vi "BuildRunScript.vi"(8 "ErrorArray":errorcluster[](array[cluster]), 11 "Bus":refnum<class "Bus.lvclass">) -> (0 "ErrorArray":errorcluster[](array[cluster]), 2 "Script":string[](array[string]), 3 "Bus":refnum<class "Bus.lvclass">)   [LabVIEW 2014, in "Bus_class.lvlib" / "Bus.lvclass"]
uses:
  Bus.lvclass
  Modules/EventModule/PublicAPI/Arguments/Broadcasts/clErrorRpt.ctl
  <vilib>/Utility/error.llb/Error Cluster From Error Code.vi
  <vilib>/ErrorRing/Error Ring.xnode
  Modules/EventModule/EventModule.lvlib
  <userlib>/NIST/NISTErrorLib/NISTErrorLib.lvlib
  Modules/PmuImpairModule/PmuImpairModule.lvlib
  Modules/NetworkImpairmentModule/NetworkImpairmentModule.lvlib
  Modules/FlagImpairModule/FlagImpairModule.lvlib
  Modules/OutputToFileModule/OutputToFileModule.lvlib
  Modules/AppModule/AppModule.lvlib
  Modules/AppPlugins/AppPluginBaseClass/AppPluginsBase.lvclass
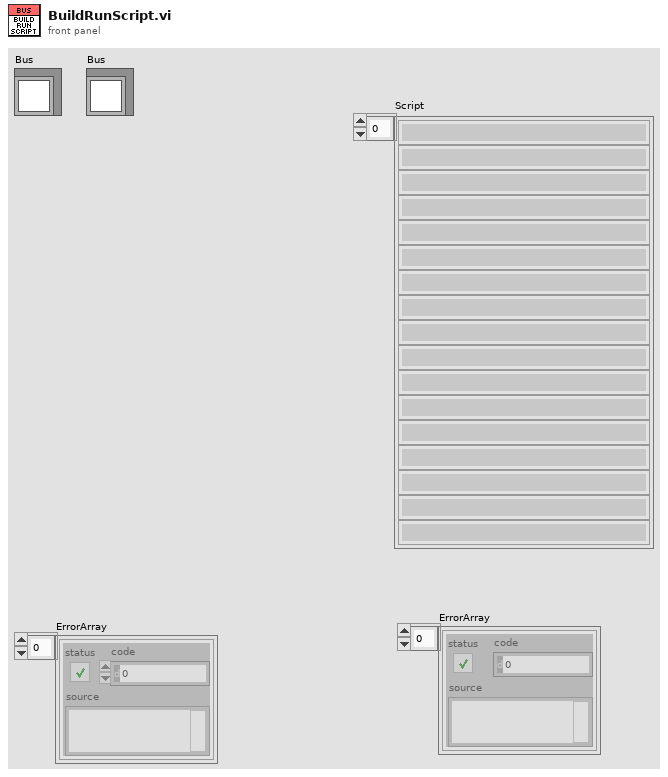
[diagram p1: front panel]
types:
  T1 = typedef "EventModule.lvlib/clErrorRpt.ctl" = cluster{"error":errorcluster, "AdditionalInfo":string}
  T2 = typedef "EventModule.lvlib/clBroadcastEvents.ctl" = cluster{"DidInit":refnum<user-event>, "StatusUpdate":refnum<user-event>, "ErrorReport":refnum<user-event>, "DidStop":refnum<user-event>, "ReadEvtConfig":refnum<user-event>, "ReadTimeArray":refnum<user-event>, "ReadEvtParams":refnum<user-event>, "GetEvtReportArray":refnum<user-event>, "ReadPathToPlugin":refnum<user-event>, "GetEvtSignal":refnum<user-event>, "ReadBusNumber":refnum<user-event>}
  T3 = typedef "PmuImpairModule.lvlib/clBroadcastEvents.ctl" = cluster{"DidInit":refnum<user-event>, "StatusUpdate":refnum<user-event>, "ErrorReport":refnum<user-event>, "DidStop":refnum<user-event>, "ImpairConfig":refnum<user-event>, "ImpairParams":refnum<user-event>, "ImpairReports":refnum<user-event>, "PathToPlugin":refnum<user-event>, "BusNumber":refnum<user-event>}
  T4 = typedef "NetworkImpairmentModule.lvlib/clBroadcastEvents.ctl" = cluster{"DidInit":refnum<user-event>, "StatusUpdate":refnum<user-event>, "ErrorReport":refnum<user-event>, "DidStop":refnum<user-event>, "ReadNetImpParams":refnum<user-event>, "ReadLossThreshold":refnum<user-event>, "GetNetworkTime":refnum<user-event>, "GetPktLoss":refnum<user-event>, "ReadPathToPlugin":refnum<user-event>}
  T5 = typedef "FlagImpairModule.lvlib/clBroadcastEvents.ctl" = cluster{"DidInit":refnum<user-event>, "StatusUpdate":refnum<user-event>, "ErrorReport":refnum<user-event>, "DidStop":refnum<user-event>, "ReadFlagImpairConfig":refnum<user-event>, "ReadPluginINIFilePath":refnum<user-event>, "ReadFlagImpairParams":refnum<user-event>, "ReadTimeArray":refnum<user-event>, "GetFlagImpairment":refnum<user-event>}
  T6 = typedef "OutputToFileModule.lvlib/clBroadcastEvents.ctl" = cluster{"DidInit":refnum<user-event>, "StatusUpdate":refnum<user-event>, "ErrorReport":refnum<user-event>, "DidStop":refnum<user-event>, "PathToPlugin":refnum<user-event>, "PmuConfig":refnum<user-event>, "OutputPath":refnum<user-event>}
  T7 = typedef "AppModule.lvlib/clBroadcastEvents.ctl" = cluster{"DidInit":refnum<user-event>, "StatusUpdate":refnum<user-event>, "ErrorReport":refnum<user-event>, "DidStop":refnum<user-event>, "PathToINI":refnum<user-event>, "InputData":refnum<user-event>, "OutputData":refnum<user-event>, "BcAppInfo":refnum<user-event>, "ConfigData":refnum<user-event>}
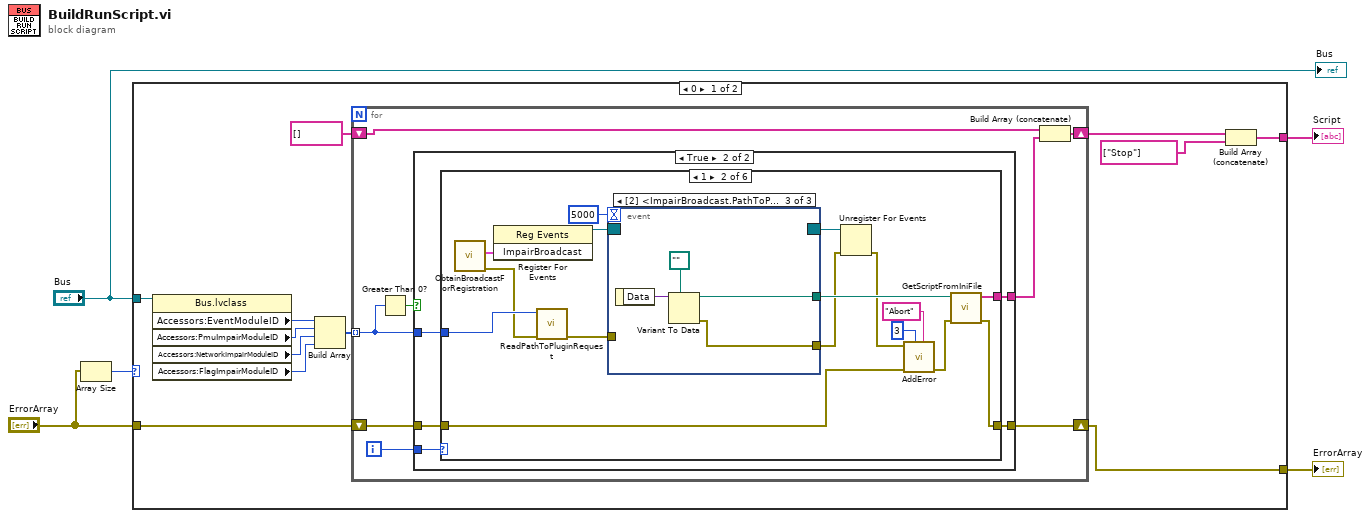
[diagram p0: block diagram]
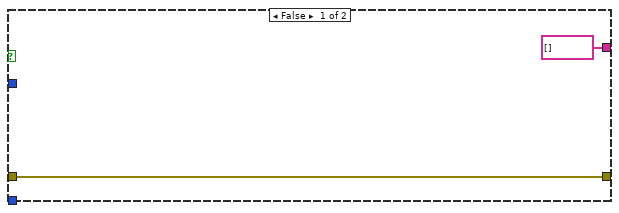
[diagram p2: hidden frame]
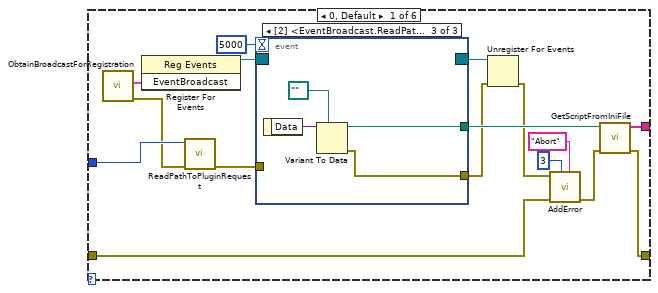
[diagram p3: hidden frame]
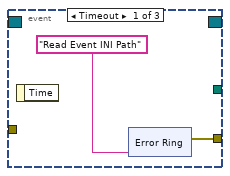
[diagram p4: hidden frame]
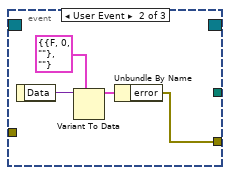
[diagram p5: hidden frame]
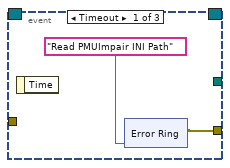
[diagram p6: hidden frame]
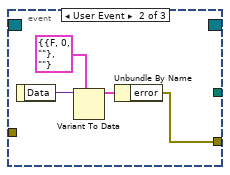
[diagram p7: hidden frame]
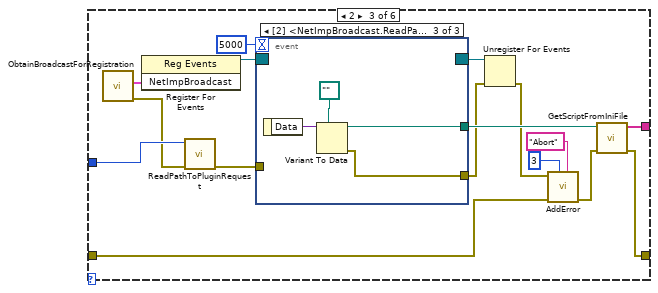
[diagram p8: hidden frame]
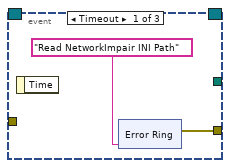
[diagram p9: hidden frame]
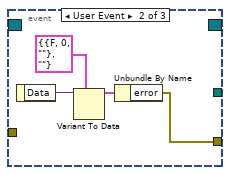
[diagram p10: hidden frame]
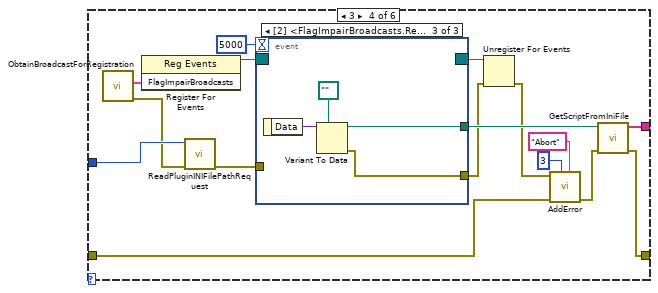
[diagram p11: hidden frame]
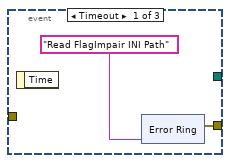
[diagram p12: hidden frame]
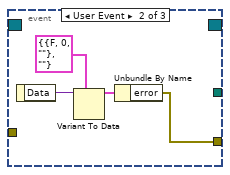
[diagram p13: hidden frame]
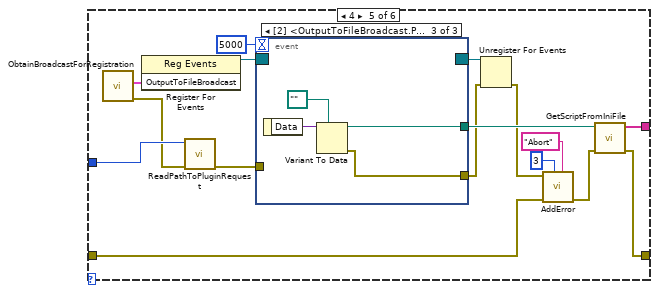
[diagram p14: hidden frame]
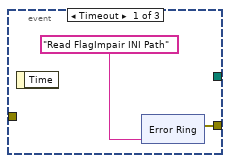
[diagram p15: hidden frame]
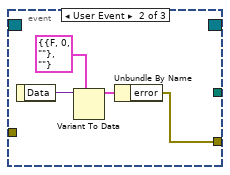
[diagram p16: hidden frame]
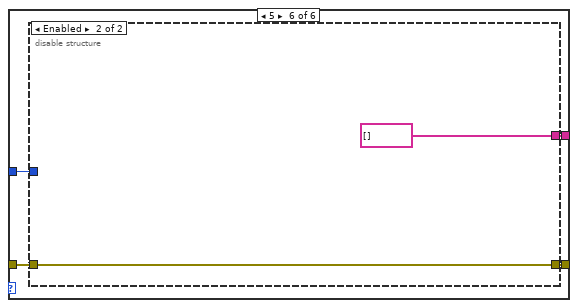
[diagram p17: hidden frame]
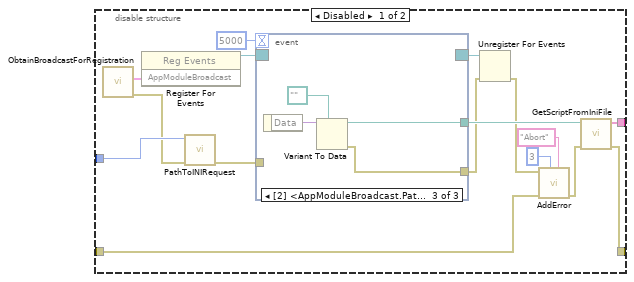
[diagram p18: hidden frame]
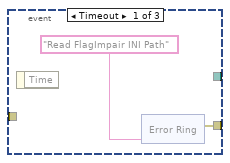
[diagram p19: hidden frame]
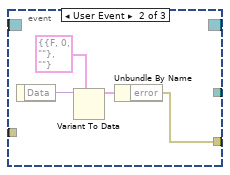
[diagram p20: hidden frame]
diagram:
  n1 = Array Size(array="ErrorArray") -> (size(s)=w5:i32)
  n2 = case shown="0" w5 {
    tunnel: "ErrorArray" -> [w10 w237]
    tunnel: [w8 w237] -> w3
    tunnel: [w17 _] -> w2
    tunnel: "Bus" -> [w6 _]
    frame 0 {
      n3 = property class="Bus.lvclass"(reference=w6) -> ("Accessors:EventModuleID"=w15:i32, "Accessors:PmuImpairModuleID"=w14:i32, "Accessors:NetworkImpairModuleID"=w13:i32, "Accessors:FlagImpairModuleID"=w12:i32)  [unwired: 1 in, 2 out]
      n4 = Build Array(w15, w14, w13, w12) -> (w11:i32[])
      n5 = for {
        tunnel: w11 -> [w18] mode=indexing
        shift-right: [w23] -> w8
        shift-left: w10 -> [w24]
        shift-right: [w21] -> w7
        shift-left: string[] [] -> [w20]
        i -> [w25]
        n6 = Greater Than 0?(x=w18) -> (x > 0?=w19:bool)
        n7 = case shown="True" w19 {
          tunnel: w25 -> [_ w32]
          tunnel: w18 -> [_ w31]
          tunnel: w24 -> [w26 w30]
          tunnel: [w26 w29] -> w23
          tunnel: [string[] [] ("Script") w28] -> w22
          frame False {
          }
          frame True {
            n8 = case shown="1" w32 {
              tunnel: w31 -> [w48 w81 w114 w147 w180 w201]
              tunnel: w30 -> [w38 w71 w104 w137 w170 w200]
              tunnel: [w37 w70 w103 w136 w169 w199] -> w29
              tunnel: [w36 w69 w102 w135 w168 w198] -> w28
              frame 0, Default {
                n9 = call "ObtainBroadcastForRegistration.vi"() -> ("error out"=w43:errorcluster, "EventBroadcast"=w47:T2)  [unwired: 10 in]
                n10 = register-events(w47) -> (reference out=w46:refnum<event-registration>)  [unwired: 2 in, 1 out]
                n11 = call "ReadPathToPluginRequest.vi"("error in (no error)"=w43, "ModuleID"=w48) -> ("error out"=w44:errorcluster)  [unwired: 9 in]
                n12 = event shown="[2] <EventBroadcast.ReadPathToPlugin>: User Event" {
                  selector: w46 -> [_ _ _]
                  dyn-events: [_ _ _] -> w35
                  timeout: 5000 -> [_ _ _]
                  tunnel: [w50 w58 w63] -> w34
                  tunnel: w44 -> [_ _ _]
                  tunnel: [_ _ w62] -> w42
                  event Timeout {
                    n13 = event-data() -> ()  [unwired: 1 in, 1 out]
                    n14 = xnode "Error Ring"("parameter 0"="Read Event INI Path") -> ("error out"=w50:errorcluster)
                  }
                  event User Event {
                    n15 = event-data() -> ("Data"=w61:variant)  [unwired: 1 in]
                    n16 = Variant To Data(type=T1 {"error"={"status"=FALSE, "code"=0, "source"=""}, "AdditionalInfo"=""} ("Cluster"), Variant=w61) -> (data=w59:T1)  [unwired: 1 in, 1 out]
                    n17 = Unbundle By Name(w59) -> ("error"=w58:errorcluster)
                  }
                  event User Event {
                    n18 = event-data() -> ("Data"=w65:variant)  [unwired: 1 in]
                    n19 = Variant To Data(type=path "", Variant=w65) -> (data=w62:path, error out=w63:errorcluster)  [unwired: 1 in]
                  }
                }
                n20 = Unregister For Events(event registration refnum=w35, error in=w34) -> (error out=w33:errorcluster)
                n21 = call <userlib>:"AddError.vi"("Severity"="Abort" ("String"), "Priority"=u8 3, "ErrorArray"=w38, "error in (no error)"=w33) -> ("ErrorArray"=w39:errorcluster[])  [unwired: 6 in, 1 out]
                n22 = call "GetScriptFromIniFile.vi"("ErrorArray"=w39, "Path"=w42) -> ("ErrorArray"=w37:errorcluster[], "Script"=w36:string[])  [unwired: 8 in]
              }
              frame 1 {
                n23 = call "ObtainBroadcastForRegistration.vi"() -> ("error out"=w76:errorcluster, "ImpairBroadcast"=w80:T3)  [unwired: 10 in]
                n24 = register-events(w80) -> (reference out=w79:refnum<event-registration>)  [unwired: 2 in, 1 out]
                n25 = call "ReadPathToPluginRequest.vi"("error in (no error)"=w76, "ModuleID"=w81) -> ("error out"=w77:errorcluster)  [unwired: 9 in]
                n26 = event shown="[2] <ImpairBroadcast.PathToPlugin>: User Event" {
                  selector: w79 -> [_ _ _]
                  dyn-events: [_ _ _] -> w68
                  timeout: 5000 -> [_ _ _]
                  tunnel: [w83 w91 w96] -> w67
                  tunnel: w77 -> [_ _ _]
                  tunnel: [_ _ w95] -> w75
                  event Timeout {
                    n27 = event-data() -> ()  [unwired: 1 in, 1 out]
                    n28 = xnode "Error Ring"("parameter 0"="Read PMUImpair INI Path") -> ("error out"=w83:errorcluster)
                  }
                  event User Event {
                    n29 = event-data() -> ("Data"=w94:variant)  [unwired: 1 in]
                    n30 = Variant To Data(type=T1 {"error"={"status"=FALSE, "code"=0, "source"=""}, "AdditionalInfo"=""} ("Cluster"), Variant=w94) -> (data=w92:T1)  [unwired: 1 in, 1 out]
                    n31 = Unbundle By Name(w92) -> ("error"=w91:errorcluster)
                  }
                  event User Event {
                    n32 = event-data() -> ("Data"=w98:variant)  [unwired: 1 in]
                    n33 = Variant To Data(type=path "", Variant=w98) -> (data=w95:path, error out=w96:errorcluster)  [unwired: 1 in]
                  }
                }
                n34 = Unregister For Events(event registration refnum=w68, error in=w67) -> (error out=w66:errorcluster)
                n35 = call <userlib>:"AddError.vi"("Severity"="Abort" ("String"), "Priority"=u8 3, "ErrorArray"=w71, "error in (no error)"=w66) -> ("ErrorArray"=w72:errorcluster[])  [unwired: 6 in, 1 out]
                n36 = call "GetScriptFromIniFile.vi"("ErrorArray"=w72, "Path"=w75) -> ("ErrorArray"=w70:errorcluster[], "Script"=w69:string[])  [unwired: 8 in]
              }
              frame 2 {
                n37 = call "ObtainBroadcastForRegistration.vi"() -> ("error out"=w109:errorcluster, "NetImpBroadcast"=w113:T4)  [unwired: 10 in]
                n38 = register-events(w113) -> (reference out=w112:refnum<event-registration>)  [unwired: 2 in, 1 out]
                n39 = call "ReadPathToPluginRequest.vi"("error in (no error)"=w109, "ModuleID"=w114) -> ("error out"=w110:errorcluster)  [unwired: 9 in]
                n40 = event shown="[2] <NetImpBroadcast.ReadPathToPlugin>: User Event" {
                  selector: w112 -> [_ _ _]
                  dyn-events: [_ _ _] -> w101
                  timeout: 5000 -> [_ _ _]
                  tunnel: [w116 w124 w129] -> w100
                  tunnel: w110 -> [_ _ _]
                  tunnel: [_ _ w128] -> w108
                  event Timeout {
                    n41 = event-data() -> ()  [unwired: 1 in, 1 out]
                    n42 = xnode "Error Ring"("parameter 0"="Read NetworkImpair INI Path") -> ("error out"=w116:errorcluster)
                  }
                  event User Event {
                    n43 = event-data() -> ("Data"=w127:variant)  [unwired: 1 in]
                    n44 = Variant To Data(type=T1 {"error"={"status"=FALSE, "code"=0, "source"=""}, "AdditionalInfo"=""} ("Cluster"), Variant=w127) -> (data=w125:T1)  [unwired: 1 in, 1 out]
                    n45 = Unbundle By Name(w125) -> ("error"=w124:errorcluster)
                  }
                  event User Event {
                    n46 = event-data() -> ("Data"=w131:variant)  [unwired: 1 in]
                    n47 = Variant To Data(type=path "", Variant=w131) -> (data=w128:path, error out=w129:errorcluster)  [unwired: 1 in]
                  }
                }
                n48 = Unregister For Events(event registration refnum=w101, error in=w100) -> (error out=w99:errorcluster)
                n49 = call <userlib>:"AddError.vi"("Severity"="Abort" ("String"), "Priority"=u8 3, "ErrorArray"=w104, "error in (no error)"=w99) -> ("ErrorArray"=w105:errorcluster[])  [unwired: 6 in, 1 out]
                n50 = call "GetScriptFromIniFile.vi"("ErrorArray"=w105, "Path"=w108) -> ("ErrorArray"=w103:errorcluster[], "Script"=w102:string[])  [unwired: 8 in]
              }
              frame 3 {
                n51 = call "ObtainBroadcastForRegistration.vi"() -> ("error out"=w142:errorcluster, "FlagImpairBroadcasts"=w146:T5)  [unwired: 10 in]
                n52 = register-events(w146) -> (reference out=w145:refnum<event-registration>)  [unwired: 2 in, 1 out]
                n53 = call "ReadPluginINIFilePathRequest.vi"("error in (no error)"=w142, "ModuleID"=w147) -> ("error out"=w143:errorcluster)  [unwired: 9 in]
                n54 = event shown="[2] <FlagImpairBroadcasts.ReadPluginINIFilePath>: User Event" {
                  selector: w145 -> [_ _ _]
                  dyn-events: [_ _ _] -> w134
                  timeout: 5000 -> [_ _ _]
                  tunnel: [w149 w157 w162] -> w133
                  tunnel: w143 -> [_ _ _]
                  tunnel: [_ _ w161] -> w141
                  event Timeout {
                    n55 = event-data() -> ()  [unwired: 1 in, 1 out]
                    n56 = xnode "Error Ring"("parameter 0"="Read FlagImpair INI Path") -> ("error out"=w149:errorcluster)
                  }
                  event User Event {
                    n57 = event-data() -> ("Data"=w160:variant)  [unwired: 1 in]
                    n58 = Variant To Data(type=T1 {"error"={"status"=FALSE, "code"=0, "source"=""}, "AdditionalInfo"=""} ("Cluster"), Variant=w160) -> (data=w158:T1)  [unwired: 1 in, 1 out]
                    n59 = Unbundle By Name(w158) -> ("error"=w157:errorcluster)
                  }
                  event User Event {
                    n60 = event-data() -> ("Data"=w164:variant)  [unwired: 1 in]
                    n61 = Variant To Data(type=path "", Variant=w164) -> (data=w161:path, error out=w162:errorcluster)  [unwired: 1 in]
                  }
                }
                n62 = Unregister For Events(event registration refnum=w134, error in=w133) -> (error out=w132:errorcluster)
                n63 = call <userlib>:"AddError.vi"("Severity"="Abort" ("String"), "Priority"=u8 3, "ErrorArray"=w137, "error in (no error)"=w132) -> ("ErrorArray"=w138:errorcluster[])  [unwired: 6 in, 1 out]
                n64 = call "GetScriptFromIniFile.vi"("ErrorArray"=w138, "Path"=w141) -> ("ErrorArray"=w136:errorcluster[], "Script"=w135:string[])  [unwired: 8 in]
              }
              frame 4 {
                n65 = call "ObtainBroadcastForRegistration.vi"() -> ("error out"=w175:errorcluster, "OutputToFileBroadcast"=w179:T6)  [unwired: 10 in]
                n66 = register-events(w179) -> (reference out=w178:refnum<event-registration>)  [unwired: 2 in, 1 out]
                n67 = call "ReadPathToPluginRequest.vi"("error in (no error)"=w175, "ModuleID"=w180) -> ("error out"=w176:errorcluster)  [unwired: 9 in]
                n68 = event shown="[2] <OutputToFileBroadcast.PathToPlugin>: User Event" {
                  selector: w178 -> [_ _ _]
                  dyn-events: [_ _ _] -> w167
                  timeout: 5000 -> [_ _ _]
                  tunnel: [w182 w190 w196] -> w166
                  tunnel: w176 -> [_ _ _]
                  tunnel: [_ _ w194] -> w174
                  event Timeout {
                    n69 = event-data() -> ()  [unwired: 1 in, 1 out]
                    n70 = xnode "Error Ring"("parameter 0"="Read FlagImpair INI Path") -> ("error out"=w182:errorcluster)
                  }
                  event User Event {
                    n71 = event-data() -> ("Data"=w193:variant)  [unwired: 1 in]
                    n72 = Variant To Data(type=T1 {"error"={"status"=FALSE, "code"=0, "source"=""}, "AdditionalInfo"=""} ("Cluster"), Variant=w193) -> (data=w191:T1)  [unwired: 1 in, 1 out]
                    n73 = Unbundle By Name(w191) -> ("error"=w190:errorcluster)
                  }
                  event User Event {
                    n74 = event-data() -> ("Data"=w197:variant)  [unwired: 1 in]
                    n75 = Variant To Data(type=path "", Variant=w197) -> (data=w194:path, error out=w196:errorcluster)  [unwired: 1 in]
                  }
                }
                n76 = Unregister For Events(event registration refnum=w167, error in=w166) -> (error out=w165:errorcluster)
                n77 = call <userlib>:"AddError.vi"("Severity"="Abort" ("String"), "Priority"=u8 3, "ErrorArray"=w170, "error in (no error)"=w165) -> ("ErrorArray"=w171:errorcluster[])  [unwired: 6 in, 1 out]
                n78 = call "GetScriptFromIniFile.vi"("ErrorArray"=w171, "Path"=w174) -> ("ErrorArray"=w169:errorcluster[], "Script"=w168:string[])  [unwired: 8 in]
              }
              frame 5 {
                n79 = disable-structure shown="Enabled" {
                  disable-tunnel: w201 -> [w217 _]
                  disable-tunnel: w200 -> [w207 w235]
                  disable-tunnel: [w206 w235] -> w199
                  disable-tunnel: [w205 string[] [] ("Script")] -> w198
                  frame Disabled {
                    n80 = call "ObtainBroadcastForRegistration.vi"() -> ("error out"=w212:errorcluster, "AppModuleBroadcast"=w216:T7)  [unwired: 10 in]
                    n81 = register-events(w216) -> (reference out=w215:refnum<event-registration>)  [unwired: 2 in, 1 out]
                    n82 = call "PathToINIRequest.vi"("error in (no error)"=w212, "ModuleID"=w217) -> ("error out"=w213:errorcluster)  [unwired: 9 in]
                    n83 = event shown="[2] <AppModuleBroadcast.PathToINI>: User Event" {
                      selector: w215 -> [_ _ _]
                      dyn-events: [_ _ _] -> w204
                      timeout: 5000 -> [_ _ _]
                      tunnel: [w219 w227 w233] -> w203
                      tunnel: w213 -> [_ _ _]
                      tunnel: [_ _ w231] -> w211
                      event Timeout {
                        n84 = event-data() -> ()  [unwired: 1 in, 1 out]
                        n85 = xnode "Error Ring"("parameter 0"="Read FlagImpair INI Path") -> ("error out"=w219:errorcluster)
                      }
                      event User Event {
                        n86 = event-data() -> ("Data"=w230:variant)  [unwired: 1 in]
                        n87 = Variant To Data(type=T1 {"error"={"status"=FALSE, "code"=0, "source"=""}, "AdditionalInfo"=""} ("Cluster"), Variant=w230) -> (data=w228:T1)  [unwired: 1 in, 1 out]
                        n88 = Unbundle By Name(w228) -> ("error"=w227:errorcluster)
                      }
                      event User Event {
                        n89 = event-data() -> ("Data"=w234:variant)  [unwired: 1 in]
                        n90 = Variant To Data(type=path "", Variant=w234) -> (data=w231:path, error out=w233:errorcluster)  [unwired: 1 in]
                      }
                    }
                    n91 = Unregister For Events(event registration refnum=w204, error in=w203) -> (error out=w202:errorcluster)
                    n92 = call <userlib>:"AddError.vi"("Severity"="Abort" ("String"), "Priority"=u8 3, "ErrorArray"=w207, "error in (no error)"=w202) -> ("ErrorArray"=w208:errorcluster[])  [unwired: 6 in, 1 out]
                    n93 = call "GetScriptFromIniFile.vi"("ErrorArray"=w208, "Path"=w211) -> ("ErrorArray"=w206:errorcluster[], "Script"=w205:string[])  [unwired: 8 in]
                  }
                  frame Enabled {
                  }
                }
              }
            }
          }
        }
        n94 = Build Array (concatenate)(w20, w22) -> (w21:string[])
      }
      n95 = Build Array (concatenate)(w7, string[] ["Stop"]) -> (w17:string[])
    }
    frame 1, Default {
    }
  }
  "ErrorArray" <- w3
  "Script" <- w2
  "Bus" <- "Bus"
